vi "WPI_I2CWrite.vi"(8 "error in (no error)":errorcluster, 9 "I2CDataToSend":u8[](array[numeric]), 10 "I2CRegister":u8, 11 "I2CDevRef":T1={"DevStatus"={"status"=FALSE, "code"=0, "source"=""}, "Device Address"=0, "Handle"=0, "I2C Bus"=enum."Invalid"} {"Device Address" format="%.0x"}) -> (0 "error out":errorcluster, 3 "I2CDevRef":T1={"DevStatus"={"status"=FALSE, "code"=0, "source"=""}, "Device Address"=0, "Handle"=0, "I2C Bus"=enum."Invalid"} {"Device Address" format="%.0x"})   [LabVIEW 2017]
doc: "Writes a byte to the I2C sensor you specify.\n\nThis software is licensed. Open the labview\\readme\\WPI Robotics Library Open Source License.txt file for more information."
uses:
  <vilib>/Rock Robotics/WPI/I2C/WPI_I2CDevRef.ctl
  <vilib>/Rock Robotics/SystemInterfaces/i2clib/i2c_bus.ctl
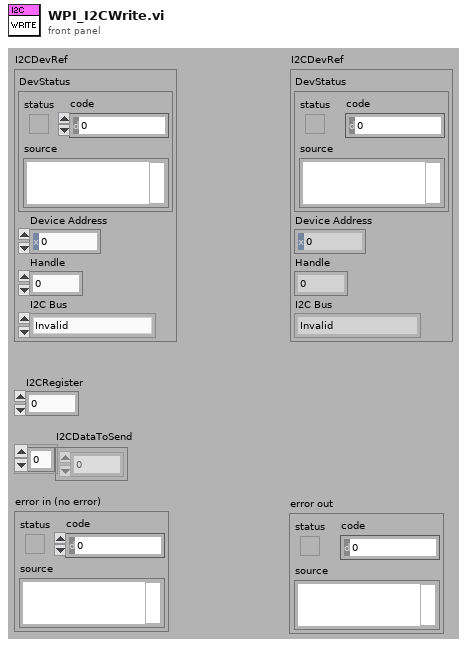
[diagram p1: front panel]
types:
  T1 = typedef "WPI_I2CDevRef.ctl" = cluster{"DevStatus":errorcluster, "Device Address":u8, "Handle":i32, "I2C Bus":T2}
  T2 = typedef "i2c_bus.ctl" = enum16{"I2C On-Board", "I2C MXP", "Invalid"}
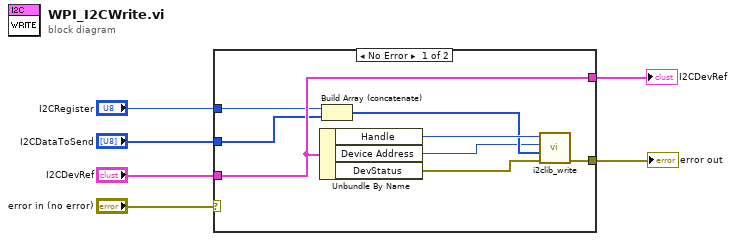
[diagram p0: block diagram]
diagram:
  n1 = case shown="No Error" "error in (no error)" {
    selector: "error in (no error)" -> [_ w16]
    tunnel: [w7 w16] -> w3
    tunnel: "I2CDevRef" -> [w14 w15]
    tunnel: [w14 w15] -> w1
    tunnel: "I2CRegister" -> [w13 _]
    tunnel: "I2CDataToSend" -> [w12 _]
    frame No Error {
      n2 = Unbundle By Name(w14) -> ("Handle"=w11:i32, "Device Address"=w8:u8, "DevStatus"=w10:errorcluster)
      n3 = Build Array (concatenate)(w13, w12) -> (w9:u8[])
      n4 = call <vilib>:"i2clib_write.vi"("error in (no error)"=w10, "send_data"=w9, "dev_addr"=w8, "I2C Reference"=w11) -> ("error out"=w7:errorcluster)  [unwired: 6 in, 1 out]
    }
    frame Error {
    }
  }
  "I2CDevRef" <- w1
  "error out" <- w3
